vi "main.vi"() -> ()   [LabVIEW 2018]
panel:
  out "Open SubVI Front Panel Indicator":bool
  in  "Open SubVI Front Panel Control":bool
  in  "Run SubVI":bool
  in  "Stop Program":bool
  in  "Select SubVI":enum16{"SubVI 1", "SubVI 2", "SubVI 3"}(ring)
  # "Option 3 from:\nhttps://knowledge.ni.com/KnowledgeArticleDetails?id=kA00Z0000019MBISA2&l=de-DE\nAdapted from:\nhttps://www.youtube.com/watch?v=jl0wTeN954A"
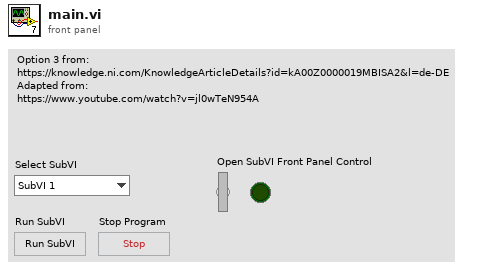
[diagram p1: front panel]
types:
  T1 = enum32{"Invalid", "Standard", "Closed", "Hidden", "Minimized", "Maximized"}
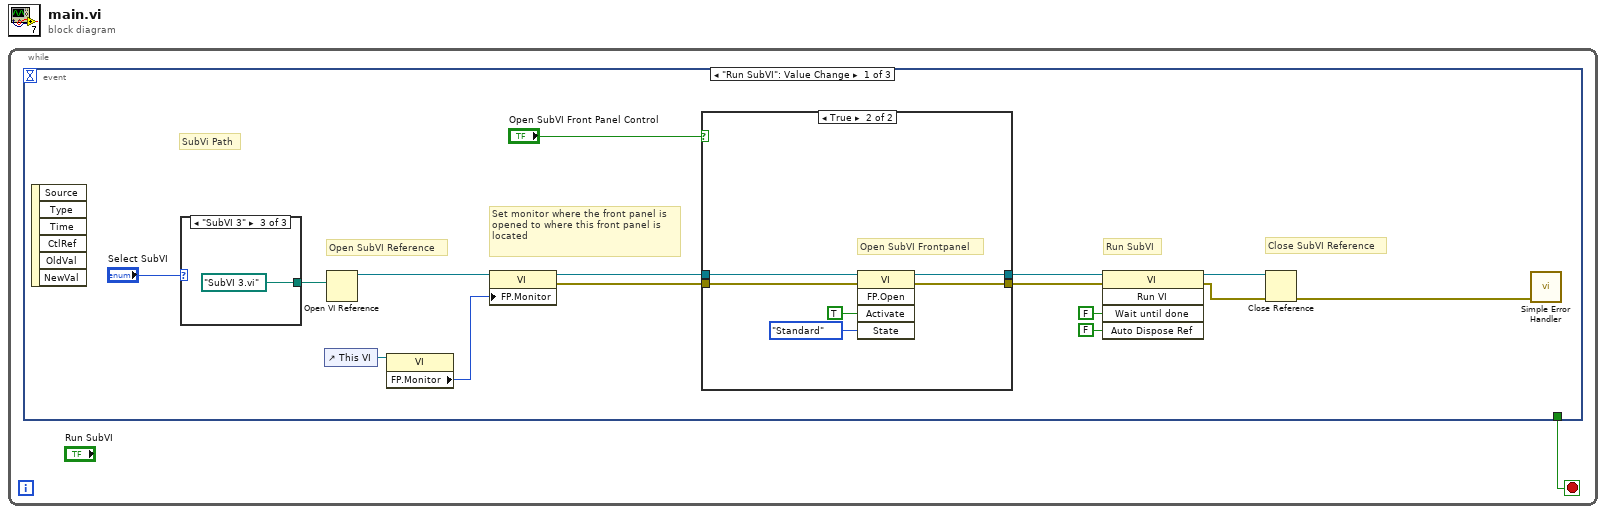
[diagram p0: block diagram]
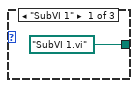
[diagram p3: hidden frame]
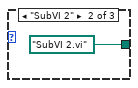
[diagram p4: hidden frame]
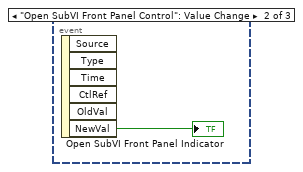
[diagram p5: hidden frame]
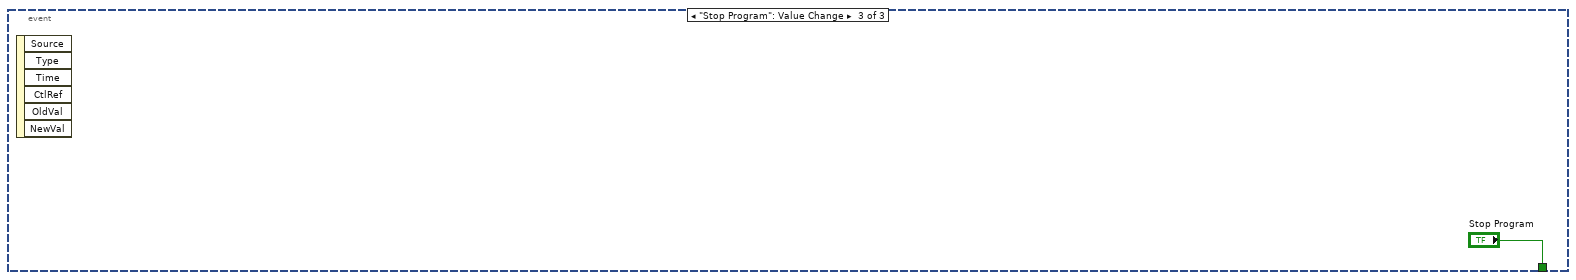
[diagram p6: hidden frame]
diagram:
  n1 = while {
    stop <- w1 stop-if-true
    n2 = event shown="[0] \"Run SubVI\": Value Change" {
      selector: _ -> [_ _ _]
      dyn-events: _ -> [_ _ _]
      timeout: _ -> [_ _ _]
      tunnel: [_ _ "Stop Program"] -> w1
      event "Run SubVI": Value Change {
        # "Set monitor where the front panel is opened to where this front panel is located"
        # "Close SubVI Reference"
        # "Run SubVI"
        # "Open SubVI Reference"
        # "SubVi Path"
        n3 = event-data() -> ()  [unwired: 1 in, 6 out]
        n4 = case shown="\"SubVI 3\"" "Select SubVI" {
          tunnel: [path "SubVI 1.vi" ("vi path") path "SubVI 2.vi" ("vi path") path "SubVI 3.vi" ("vi path")] -> w16
          frame "SubVI 1" {
          }
          frame "SubVI 2" {
          }
          frame "SubVI 3" {
          }
        }
        n5 = control-ref of="This VI"() -> (w3:refnum<vi>)
        n6 = Open VI Reference(vi path=w16) -> (vi reference=w4:refnum<vi>)  [unwired: 5 in, 1 out]
        n7 = property class="VI"(reference=w3) -> ("FP.Monitor"=w2:u16)  [unwired: 1 in, 2 out]
        n8 = property class="VI"(reference=w4, "FP.Monitor"=w2) -> (reference out=w5:refnum<vi>, error out=w6:errorcluster)  [unwired: 1 in]
        n9 = case shown="True" "Open SubVI Front Panel Control" {
          tunnel: [w17 w24] -> w15
          tunnel: [w18 w23] -> w14
          tunnel: w5 -> [w17 w22]
          tunnel: w6 -> [w18 w21]
          frame False {
          }
          frame True {
            # "Open SubVI Frontpanel"
            n10 = invoke class="VI" method="FP.Open"(reference=w22, error in=w21, "Activate"=TRUE ("Activate?"), "State"=T1."Standard") -> (reference out=w24:refnum<vi>, error out=w23:errorcluster)  [unwired: 1 in, 3 out]
          }
        }
        n11 = invoke class="VI" method="Run VI"(reference=w15, error in=w14, "Wait until done"=FALSE ("Wait Until Done"), "Auto Dispose Ref"=FALSE ("Auto Dispose Reference")) -> (reference out=w13:refnum<vi>, error out=w12:errorcluster)  [unwired: 1 in, 3 out]
        n12 = Close Reference(reference=w13, error in (no error)=w12) -> (error out=w8:errorcluster)
        n13 = call <vilib>:"Simple Error Handler.vi"("error in (no error)"=w8) -> ()  [unwired: 4 in, 5 out]
      }
      event "Open SubVI Front Panel Control": Value Change {
        n14 = event-data() -> ("NewVal"=→"Open SubVI Front Panel Indicator":bool)  [unwired: 1 in, 5 out]
      }
      event "Stop Program": Value Change {
        n15 = event-data() -> ()  [unwired: 1 in, 6 out]
      }
    }
  }
